vi "14_TEST.vi"() -> ()   [LabVIEW 2020]
uses:
  <instrlib>/Agilent B2900 Series/Agilent B2900 Series.lvlib
panel:
  in  "Time interval between iterations (seconds)":dbl
  out "XY Graph":cluster{"X":dbl[], "Y":dbl[]}[](graph)
  out "Waveform Chart":dbl(graph)
  out "Measured Output Value":dbl
  in  "SELECT DEVICE":refnum<visa-resource-name>="USB0::0x0957::0x8E18::MY51140695::INSTR"
  out "Resolution":dbl format="%#_6f"
  out "Instantaneous Input Value":dbl format="%#_6f"
  in  "Final Value":dbl
  in  "Initial Value":dbl
  in  "Steps":dbl
  in  "Measure (OUTPUT)":enum16{"Voltage", "Current"}(ring)
  in  "Source":enum16{"Voltage", "Current"}(ring)
  in  "Channel":u16(ring) items=["1", "2"]
  # "(INPUT)"
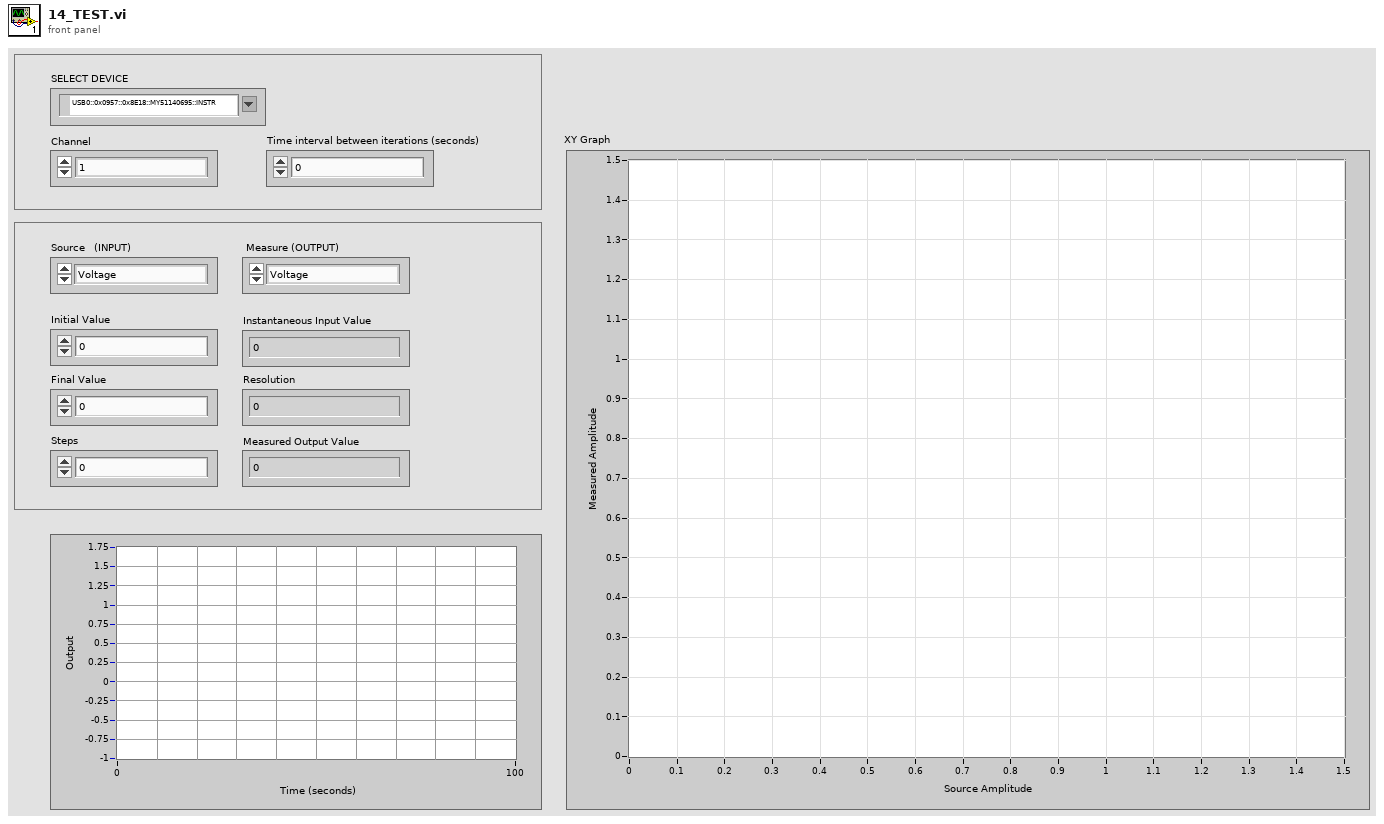
[diagram p1: front panel]
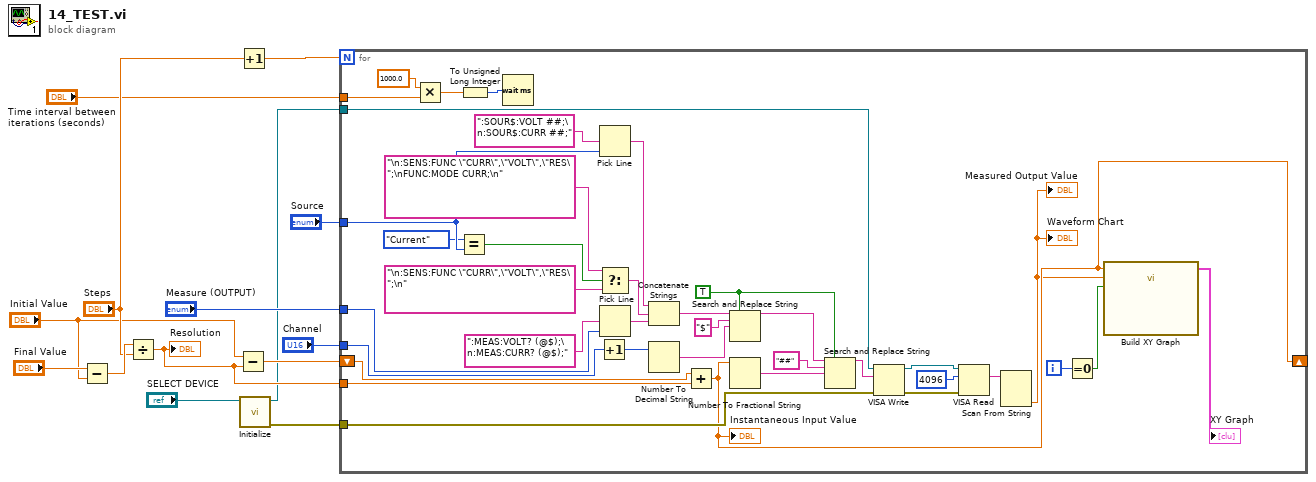
[diagram p0: block diagram]
diagram:
  n1 = Subtract(x="Final Value", y="Initial Value") -> (x-y=w9:dbl)
  n2 = Divide(x=w9, y="Steps") -> (x/y=w8:dbl)
  "Resolution" <- w8
  n3 = Subtract(x="Initial Value", y=w8) -> (x-y=w10:dbl)
  n4 = Increment(x="Steps") -> (x+1=w6:dbl)
  n5 = call <instrlib>:"Initialize.vi"("VISA resource name"="SELECT DEVICE") -> ("error out"=w2:errorcluster, "VISA resource name out"=w3:refnum<visa-resource-name>)  [unwired: 9 in]
  n6 = for {
    N: w6 -> [_]
    tunnel: "Channel" -> [w51]
    tunnel: "Source" -> [w36]
    tunnel: "Measure (OUTPUT)" -> [w49]
    tunnel: w8 -> [w37]
    shift-right: [w24] -> _
    shift-left: w10 -> [w38]
    tunnel: w3 -> [w27]
    tunnel: w2 -> [w26]
    tunnel: "Time interval between iterations (seconds)" -> [w18]
    i -> [w21]
    w40 = TRUE ("replace all? (F)")
    n7 = Multiply(x=1000.0, y=w18) -> (x*y=w15:dbl)
    n8 = Equal?(x=enum16{"Voltage", "Current"}."Current", y=w36) -> (x = y?=w33:bool)
    n9 = To Unsigned Long Integer(number=w15) -> (unsigned 32bit integer=w16:u32)
    n10 = Wait (ms)(milliseconds to wait=w16) -> ()  [unwired: 1 out]
    n11 = Increment(x=w51) -> (x+1=w44:u16)
    n12 = Pick Line(multi-line string=":SOUR$:VOLT ##;\n:SOUR$:CURR ##;", line index=w36) -> (output string=w47:string)  [unwired: 1 in]
    n13 = Select(t="\n:SENS:FUNC \"CURR\",\"VOLT\",\"RES\";\nFUNC:MODE CURR;\n" ("string"), s=w33, f="\n:SENS:FUNC \"CURR\",\"VOLT\",\"RES\";\n") -> (s? t:f=w31:string)
    n14 = Pick Line(multi-line string=":MEAS:VOLT? (@$);\n:MEAS:CURR? (@$);", line index=w49) -> (output string=w48:string)  [unwired: 1 in]
    n15 = Concatenate Strings(w47, w31, w48) -> (w46:string)
    n16 = Number To Decimal String(number=w44) -> (decimal integer string=w43:string)  [unwired: 1 in]
    n17 = Add(x=w38, y=w37) -> (x+y=w24:dbl)
    "Instantaneous Input Value" <- w24
    n18 = Search and Replace String(replace all?=w40, input string=w46, search string="$", replace string=w43) -> (result string=w42:string)  [unwired: 4 in, 3 out]
    n19 = Number To Fractional String(number=w24) -> (F-format string=w39:string)  [unwired: 3 in]
    n20 = Search and Replace String(replace all?=w40, input string=w42, search string="##", replace string=w39) -> (result string=w19:string)  [unwired: 4 in, 3 out]
    n21 = VISA Write(VISA resource name=w27, write buffer=w19, error in (no error)=w26) -> (VISA resource name out=w28:refnum<visa-resource-name>, error out=w29:errorcluster)  [unwired: 1 out]
    n22 = VISA Read(VISA resource name=w28, byte count=u32 4096, error in (no error)=w29) -> (read buffer=w25:string)  [unwired: 3 out]
    n23 = Scan From String(input string=w25) -> (output 1=w23:dbl)  [unwired: 4 in, 3 out]
    "Measured Output Value" <- w23
    "Waveform Chart" <- w23
    n24 = Equal To 0?(x=w21) -> (x = 0?=w20:bool)
    n25 = call "Build XY Graph"("Reset"=w20, "Y Input"=w23, "X Input"=w24) -> ("XY Graph"=→"XY Graph":cluster{"X":dbl[], "Y":dbl[]}[])  [unwired: 7 in, 1 out]
  }
